vi "GUSID Hash Thing.vi"() -> (3 "String":string)   [LabVIEW 2013]
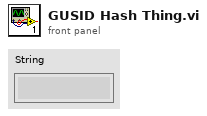
[diagram p1: front panel]
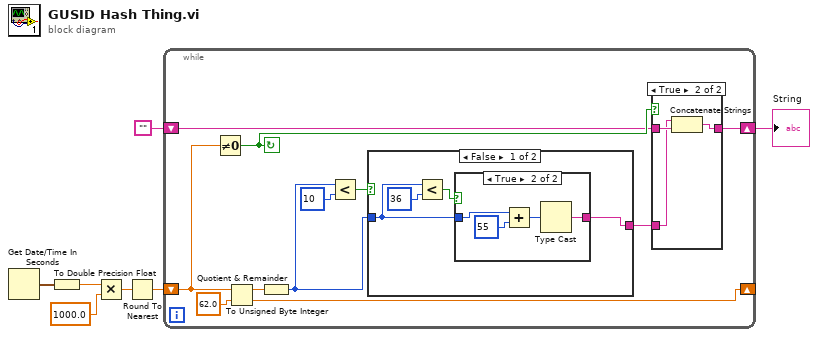
[diagram p0: block diagram]
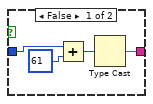
[diagram p3: hidden frame]
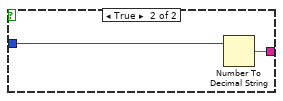
[diagram p4: hidden frame]
diagram:
  n1 = Get Date/Time In Seconds() -> (seconds since 1Jan1904=w7:timestamp)
  n2 = To Double Precision Float(number=w7) -> (double precision float=w6:dbl)
  n3 = Multiply(x=w6, y=1000.0) -> (x*y=w3:dbl)
  n4 = Round To Nearest(number=w3) -> (nearest integer value=w4:dbl)
  n5 = while {
    shift-right: [w16] -> _
    shift-left: w4 -> [w18]
    shift-right: [w8] -> w1
    shift-left: "" -> [w10]
    stop <- w11 continue-if-true
    n6 = Not Equal To 0?(x=w18) -> (x != 0?=w11:bool)
    n7 = Quotient & Remainder(x=w18, y=62.0) -> (x-y*floor(x/y)=w13:dbl, floor(x/y)=w16:dbl)
    n8 = To Unsigned Byte Integer(number=w13) -> (unsigned 8bit integer=w12:u8)
    n9 = Less?(x=w12, y=u8 10) -> (x < y?=w15:bool)
    n10 = case shown="False" w15 {
      tunnel: w12 -> [w24 w36]
      tunnel: [w23 w35] -> w9
      frame False {
        n11 = Less?(x=w24, y=u8 36) -> (x < y?=w25:bool)
        n12 = case shown="True" w25 {
          tunnel: w24 -> [w30 w34]
          tunnel: [w27 w31] -> w23
          frame False {
            n13 = Add(x=w30, y=u8 61) -> (x+y=w28:u8)
            n14 = Type Cast(x=w28) -> (*(type *) &x=w27:string)  [unwired: 1 in]
          }
          frame True {
            n15 = Add(x=w34, y=u8 55) -> (x+y=w32:u8)
            n16 = Type Cast(x=w32) -> (*(type *) &x=w31:string)  [unwired: 1 in]
          }
        }
      }
      frame True {
        n17 = Number To Decimal String(number=w36) -> (decimal integer string=w35:string)  [unwired: 1 in]
      }
    }
    n18 = case shown="True" w11 {
      tunnel: w10 -> [w19 w21]
      tunnel: w9 -> [_ w20]
      tunnel: [w19 w22] -> w8
      frame False {
      }
      frame True {
        n19 = Concatenate Strings(w20, w21) -> (w22:string)
      }
    }
  }
  "String" <- w1
